vi "S7.vi"   [LabVIEW 2020]
uses:
  S7Ref.vi
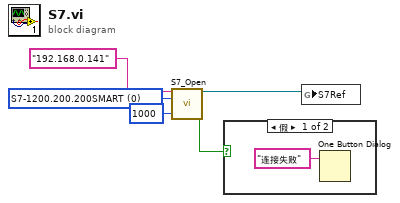
[diagram p0: block diagram]
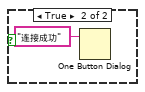
[diagram p2: hidden frame]
diagram:
  w4 = u8 0 items=["S7-1200.200.200SMART"=0, "S7-300"=2, "S7-400"=3] ("PLC 系列")
  n1 = call "S7_Open.vi"("IP 地址"="192.168.0.141", "PLC 系列"=w4, "超时（MS）"=1000) -> ("TCP"=w2:refnum<k5>, "连接"=w1:bool)  [unwired: 10 in, 1 out]
  n2 = case shown="假" w1 {
    frame False {
      n3 = One Button Dialog(message="连接失败" ("消息")) -> ()  [unwired: 1 in, 1 out]
    }
    frame True {
      n4 = One Button Dialog(message="连接成功" ("消息")) -> ()  [unwired: 1 in, 1 out]
    }
  }
  n5 = global write "S7Ref.vi" "S7Ref"(w2) -> ()
